vi "test-timer-all.vi"() -> (3 "ALL TESTS PASSED":bool)   [LabVIEW 2019]
uses:
  <vilib>/Rock Robotics/WPI/ThirdParty/JAS_Junk/TrajLib/Trajectory_Library.lvlib
panel:
  out "Expired 2":bool
  out "Expired":bool
  out "T2 After Start":dbl
  out "Passed 2":bool
  out "T1 After Stop":dbl
  out "T1 After Start":dbl
  out "Passed 0A":bool
  out "Passed 0":bool
  out "T0 - Diff = 5.0":dbl
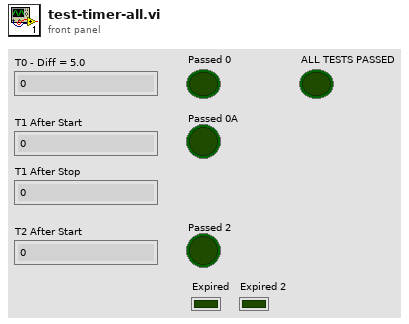
[diagram p1: front panel]
types:
  T1 = typedef "Trajectory_Library.lvlib/TIMER.ctl" = cluster{"StartTime":dbl, "Accumulated TIme":dbl, "Running":bool, "semaphore":T2}
  T2 = typedef "Semaphore RefNum" = refnum<k1>
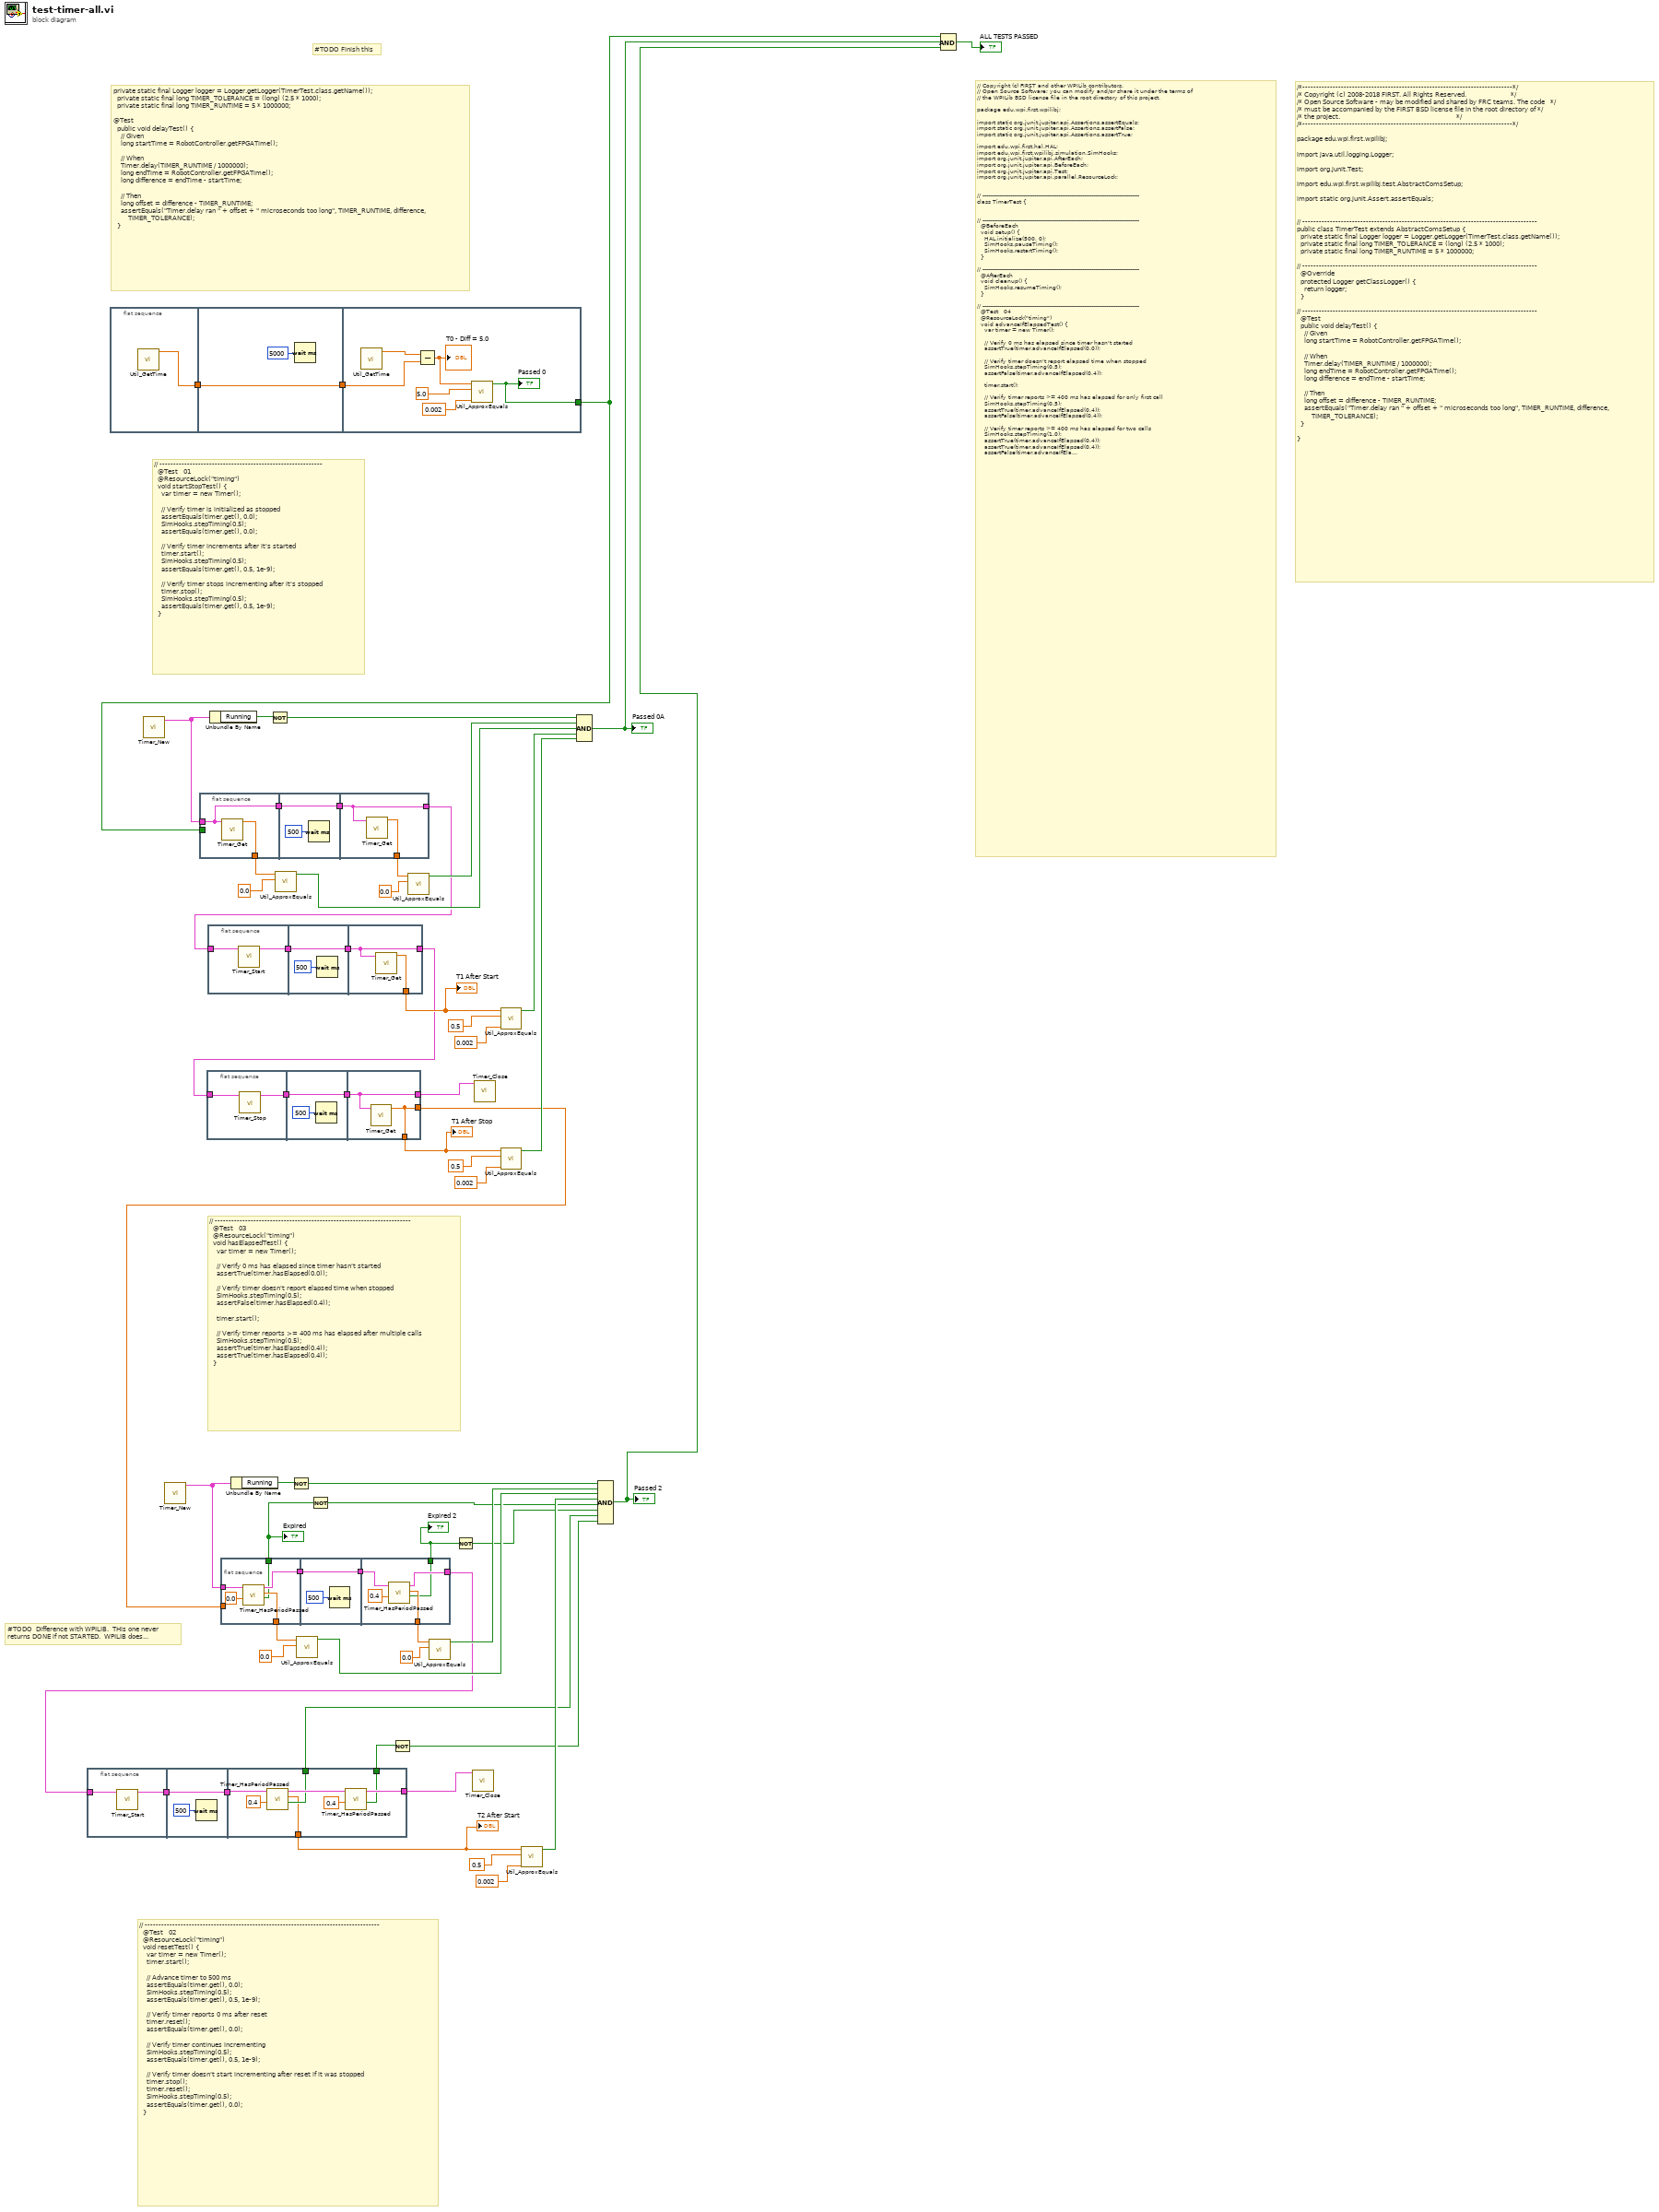
[diagram p0: block diagram]
diagram:
  # "#TODO Finish this"
  # "// -------------------------------------------------------------------------------------\n  @Test   02\n  @ResourceLock(\"timing\")\n  void resetTest() {\n    var timer = new Timer();\n    timer.start();\n\n    // Advance timer to 500 ms\n    assertEquals(timer.get(), 0.0);\n    SimHooks.stepTiming(0.5);\n    assertEquals(timer.get(), 0.5, 1e-9);\n\n    // Verify timer reports 0 ms after reset\n    timer.reset();\n    assertEquals(timer.get(), 0.0);\n\n    // Verify timer continues incrementing\n    SimHooks.stepTiming(0.5);\n    assertEquals(timer.get(), 0.5, 1e-9);\n\n    // Verify timer doesn't start incrementing after reset if it was stopped\n    timer.stop();\n    timer.reset();\n    SimHooks.stepTiming(0.5);\n    assertEquals(timer.get(), 0.0);\n  }"
  # "#TODO  Difference with WPILIB.  THis one never\nreturns DONE if not STARTED.  WPILIB does..."
  # "// -----------------------------------------------------------------------\n  @Test   03\n  @ResourceLock(\"timing\")\n  void hasElapsedTest() {\n    var timer = new Timer();\n\n    // Verify 0 ms has elapsed since timer hasn't started\n    assertTrue(timer.hasElapsed(0.0));\n\n    // Verify timer doesn't report elapsed time when stopped\n    SimHooks.stepTiming(0.5);\n    assertFalse(timer.hasElapsed(0.4));\n\n    timer.start();\n\n    // Verify timer reports >= 400 ms has elapsed after multiple calls\n    SimHooks.stepTiming(0.5);\n    assertTrue(timer.hasElapsed(0.4));\n    assertTrue(timer.hasElapsed(0.4));\n  }"
  # "// -----------------------------------------------------------\n  @Test   01\n  @ResourceLock(\"timing\")\n  void startStopTest() {\n    var timer = new Timer();\n\n    // Verify timer is initialized as stopped\n    assertEquals(timer.get(), 0.0);\n    SimHooks.stepTiming(0.5);\n    assertEquals(timer.get(), 0.0);\n\n    // Verify timer increments after it's started\n    timer.start();\n    SimHooks.stepTiming(0.5);\n    assertEquals(timer.get(), 0.5, 1e-9);\n\n    // Verify timer stops incrementing after it's stopped\n    timer.stop();\n    SimHooks.stepTiming(0.5);\n    assertEquals(timer.get(), 0.5, 1e-9);\n  }"
  # "/*----------------------------------------------------------------------------*/\n/* Copyright (c) 2008-2018 FIRST. All Rights Reserved.                        */\n/* Open Source Software - may be modified and shared by FRC teams. The code   */\n/* must be accompanied by the FIRST BSD license file in the root directory of */\n/* the project.                                                               */\n/*----------------------------------------------------------------------------*/\n\npackage edu.wpi.first.wpilibj;\n\nimport java.util.logging.Logger;\n\nimport org.junit.Test;\n\nimport edu.wpi.first.wpilibj.test.AbstractComsSetup;\n\nimport static org.junit.Assert.assertEquals;\n\n\n// -------------------------------------------------------------------------------------\npublic class TimerTest extends AbstractComsSetup {\n  private static final Logger logger = Logger.getLogger(TimerTest.class.getName());\n  private static final long TIMER_TOLERANCE = (long) (2.5 * 1000);\n  private static final long TIMER_RUNTIME = 5 * 1000000;\n\n// -------------------------------------------------------------------------------------\n  @Override\n  protected Logger getClassLogger() {\n    return logger;\n  }\n\n// -------------------------------------------------------------------------------------\n  @Test\n  public void delayTest() {\n    // Given\n    long startTime = RobotController.getFPGATime();\n\n    // When\n    Timer.delay(TIMER_RUNTIME / 1000000);\n    long endTime = RobotController.getFPGATime();\n    long difference = endTime - startTime;\n\n    // Then\n    long offset = difference - TIMER_RUNTIME;\n    assertEquals(\"Timer.delay ran \" + offset + \" microseconds too long\", TIMER_RUNTIME, difference,\n        TIMER_TOLERANCE);\n  }\n\n}"
  # "// Copyright (c) FIRST and other WPILib contributors.\n// Open Source Software; you can modify and/or share it under the terms of\n// the WPILib BSD license file in the root directory of this project.\n\npackage edu.wpi.first.wpilibj;\n\nimport static org.junit.jupiter.api.Assertions.assertEquals;\nimport static org.junit.jupiter.api.Assertions.assertFalse;\nimport static org.junit.jupiter.api.Assertions.assertTrue;\n\nimport edu.wpi.first.hal.HAL;\nimport edu.wpi.first.wpilibj.simulation.SimHooks;\nimport org.junit.jupiter.api.AfterEach;\nimport org.junit.jupiter.api.BeforeEach;\nimport org.junit.jupiter.api.Test;\nimport org.junit.jupiter.api.parallel.ResourceLock;\n\n\n// -------------------------------------------------------------------------------------\nclass TimerTest {\n\n\n// -------------------------------------------------------------------------------------\n  @BeforeEach\n  void setup() {\n    HAL.initialize(500, 0);\n    SimHooks.pauseTiming();\n    SimHooks.restartTiming();\n  }\n\n// -------------------------------------------------------------------------------------\n  @AfterEach\n  void cleanup() {\n    SimHooks.resumeTiming();\n  }\n\n// -------------------------------------------------------------------------------------\n  @Test   04\n  @ResourceLock(\"timing\")\n  void advanceIfElapsedTest() {\n    var timer = new Timer();\n\n    // Verify 0 ms has elapsed since timer hasn't started\n    assertTrue(timer.advanceIfElapsed(0.0));\n\n    // Verify timer doesn't report elapsed time when stopped\n    SimHooks.stepTiming(0.5);\n    assertFalse(timer.advanceIfElapsed(0.4));\n\n    timer.start();\n\n    // Verify timer reports >= 400 ms has elapsed for only first call\n    SimHooks.stepTiming(0.5);\n    assertTrue(timer.advanceIfElapsed(0.4));\n    assertFalse(timer.advanceIfElapsed(0.4));\n\n    // Verify timer reports >= 400 ms has elapsed for two calls\n    SimHooks.stepTiming(1.0);\n    assertTrue(timer.advanceIfElapsed(0.4));\n    assertTrue(timer.advanceIfElapsed(0.4));\n    assertFalse(timer.advanceIfElapsed(0.4));\n  }\n\n// -------------------------------------------------------------------------------------\n  @Test   05\n  @ResourceLock(\"timing\")\n  void getFPGATimestampTest() {\n    double start = Timer.getFPGATimestamp();\n    SimHooks.stepTiming(0.5);\n    double end = Timer.getFPGATimestamp();\n    assertEquals(start + 0.5, end, 1e-9);\n\n\n  }\n}"
  # "private static final Logger logger = Logger.getLogger(TimerTest.class.getName());\n  private static final long TIMER_TOLERANCE = (long) (2.5 * 1000);\n  private static final long TIMER_RUNTIME = 5 * 1000000;\n\n@Test\n  public void delayTest() {\n    // Given\n    long startTime = RobotController.getFPGATime();\n\n    // When\n    Timer.delay(TIMER_RUNTIME / 1000000);\n    long endTime = RobotController.getFPGATime();\n    long difference = endTime - startTime;\n\n    // Then\n    long offset = difference - TIMER_RUNTIME;\n    assertEquals(\"Timer.delay ran \" + offset + \" microseconds too long\", TIMER_RUNTIME, difference,\n        TIMER_TOLERANCE);\n  }"
  n1 = flat-sequence {
    tunnel: w19 -> [w61]
    tunnel: [w60] -> w29
    tunnel: [w62] -> w28
    tunnel: w29 -> [w62]
    tunnel: [w64] -> w17
    tunnel: w28 -> [w71]
    tunnel: [w69] -> w5
    tunnel: [w66] -> w8
    tunnel: [w65] -> w7
    frame #0 {
      n2 = call <vilib>:"Timer_Start.vi"("in Timer"=w61) -> ("out Timer"=w60:T1)  [unwired: 10 in]
    }
    frame #1 {
      n3 = Wait (ms)(milliseconds to wait=u32 500) -> ()  [unwired: 1 out]
    }
    frame #2 {
      n4 = call <vilib>:"Timer_HasPeriodPassed.vi"("Period"=0.4, "in Timer"=w71) -> ("Expired"=w66:bool, "CurrentTImer"=w64:dbl, "out Timer"=w70:T1)  [unwired: 7 in]
      n5 = call <vilib>:"Timer_HasPeriodPassed.vi"("Period"=0.4, "in Timer"=w70) -> ("Expired"=w65:bool, "out Timer"=w69:T1)  [unwired: 7 in, 1 out]
    }
  }
  n6 = flat-sequence {
    tunnel: [w72] -> w59
    tunnel: [w73] -> w58
    tunnel: w59 -> [w73]
    tunnel: w58 -> [w79]
    tunnel: [w75] -> w2
    frame #0 {
      n7 = call <vilib>:"Util_GetTime.vi"() -> ("FPGA_Time_Seconds"=w72:dbl)  [unwired: 10 in, 1 out]
    }
    frame #1 {
      n8 = Wait (ms)(milliseconds to wait=u32 5000) -> ()  [unwired: 1 out]
    }
    frame #2 {
      n9 = call <vilib>:"Util_GetTime.vi"() -> ("FPGA_Time_Seconds"=w80:dbl)  [unwired: 10 in, 1 out]
      n10 = Subtract(x=w80, y=w79) -> (x-y=w78:dbl)
      "T0 - Diff = 5.0" <- w78
      n11 = call "Util_ApproxEquals.vi"("Tolerance"=0.002, "Value 2"=5.0, "Value 1"=w78) -> ("ApproxEquals"=w75:bool)  [unwired: 8 in]
      "Passed 0" <- w75
    }
  }
  n12 = call <vilib>:"Timer_New.vi"() -> ("TIMER"=w55:T1)  [unwired: 11 in]
  n13 = call <vilib>:"Timer_New.vi"() -> ("TIMER"=w25:T1)  [unwired: 11 in]
  n14 = flat-sequence {
    tunnel: w55 -> [w81]
    tunnel: [w82] -> w53
    tunnel: [w81] -> w47
    tunnel: w2 -> [_]
    tunnel: [w83] -> w48
    tunnel: w47 -> [w83]
    tunnel: [w86] -> w54
    tunnel: w48 -> [w85]
    tunnel: [w85] -> w46
    frame #0 {
      n15 = call <vilib>:"Timer_Get.vi"("TIMER"=w81) -> ("CurrentTImer"=w82:dbl)  [unwired: 10 in]
    }
    frame #1 {
      n16 = Wait (ms)(milliseconds to wait=u32 500) -> ()  [unwired: 1 out]
    }
    frame #2 {
      n17 = call <vilib>:"Timer_Get.vi"("TIMER"=w85) -> ("CurrentTImer"=w86:dbl)  [unwired: 10 in]
    }
  }
  n18 = flat-sequence {
    tunnel: [w87] -> w39
    tunnel: w37 -> [w88]
    tunnel: [w89] -> w38
    tunnel: w39 -> [w89]
    tunnel: [w91] -> w33
    tunnel: w38 -> [w92]
    tunnel: [w92] -> w32
    tunnel: [w91] -> w14
    frame #0 {
      n19 = call <vilib>:"Timer_Stop.vi"("in Timer"=w88) -> ("out Timer"=w87:T1)  [unwired: 10 in]
    }
    frame #1 {
      n20 = Wait (ms)(milliseconds to wait=u32 500) -> ()  [unwired: 1 out]
    }
    frame #2 {
      n21 = call <vilib>:"Timer_Get.vi"("TIMER"=w92) -> ("CurrentTImer"=w91:dbl)  [unwired: 10 in]
    }
  }
  n22 = flat-sequence {
    tunnel: w46 -> [w94]
    tunnel: [w93] -> w44
    tunnel: [w95] -> w45
    tunnel: w44 -> [w95]
    tunnel: [w98] -> w42
    tunnel: w45 -> [w97]
    tunnel: [w97] -> w37
    frame #0 {
      n23 = call <vilib>:"Timer_Start.vi"("in Timer"=w94) -> ("out Timer"=w93:T1)  [unwired: 10 in]
    }
    frame #1 {
      n24 = Wait (ms)(milliseconds to wait=u32 500) -> ()  [unwired: 1 out]
    }
    frame #2 {
      n25 = call <vilib>:"Timer_Get.vi"("TIMER"=w97) -> ("CurrentTImer"=w98:dbl)  [unwired: 10 in]
    }
  }
  n26 = Unbundle By Name(w55) -> ("Running"=w57:bool)
  n27 = flat-sequence {
    tunnel: w25 -> [w102]
    tunnel: [w103] -> w24
    tunnel: [w100] -> w31
    tunnel: w14 -> [_]
    tunnel: [w99] -> w10
    tunnel: [w104] -> w30
    tunnel: w31 -> [w104]
    tunnel: w30 -> [w110]
    tunnel: [w109] -> w19
    tunnel: [w107] -> w13
    tunnel: [w106] -> w12
    frame #0 {
      n28 = call <vilib>:"Timer_HasPeriodPassed.vi"("Period"=0.0, "in Timer"=w102) -> ("Expired"=w99:bool, "CurrentTImer"=w103:dbl, "out Timer"=w100:T1)  [unwired: 7 in]
    }
    frame #1 {
      n29 = Wait (ms)(milliseconds to wait=u32 500) -> ()  [unwired: 1 out]
    }
    frame #2 {
      n30 = call <vilib>:"Timer_HasPeriodPassed.vi"("Period"=0.4, "in Timer"=w110) -> ("Expired"=w106:bool, "CurrentTImer"=w107:dbl, "out Timer"=w109:T1)  [unwired: 7 in]
    }
  }
  n31 = Unbundle By Name(w25) -> ("Running"=w27:bool)
  n32 = Not(x=w57) -> (.not. x?=w56:bool)
  n33 = call "Util_ApproxEquals.vi"("Value 2"=0.0, "Value 1"=w53) -> ("ApproxEquals"=w49:bool)  [unwired: 9 in]
  n34 = Not(x=w27) -> (.not. x?=w26:bool)
  n35 = call "Util_ApproxEquals.vi"("Value 2"=0.0, "Value 1"=w24) -> ("ApproxEquals"=w20:bool)  [unwired: 9 in]
  n36 = Not(x=w10) -> (.not. x?=w11:bool)
  n37 = Not(x=w7) -> (.not. x?=w6:bool)
  n38 = call "Util_ApproxEquals.vi"("Value 2"=0.0, "Value 1"=w54) -> ("ApproxEquals"=w50:bool)  [unwired: 9 in]
  n39 = call "Util_ApproxEquals.vi"("Value 2"=0.0, "Value 1"=w13) -> ("ApproxEquals"=w21:bool)  [unwired: 9 in]
  n40 = Not(x=w12) -> (.not. x?=w9:bool)
  n41 = call <vilib>:"Timer_Close.vi"("TIMER"=w5) -> ()  [unwired: 11 in]
  n42 = call <vilib>:"Timer_Close.vi"("TIMER"=w32) -> ()  [unwired: 11 in]
  n43 = call "Util_ApproxEquals.vi"("Tolerance"=0.002, "Value 2"=0.5, "Value 1"=w42) -> ("ApproxEquals"=w41:bool)  [unwired: 8 in]
  n44 = call "Util_ApproxEquals.vi"("Tolerance"=0.002, "Value 2"=0.5, "Value 1"=w33) -> ("ApproxEquals"=w34:bool)  [unwired: 8 in]
  n45 = call "Util_ApproxEquals.vi"("Tolerance"=0.002, "Value 2"=0.5, "Value 1"=w17) -> ("ApproxEquals"=w16:bool)  [unwired: 8 in]
  n46 = Compound Arithmetic op=AND(w56, w50, w49, w41, w34) -> (w3:bool)
  "Passed 0A" <- w3
  n47 = Compound Arithmetic op=AND(w26, w21, w20, w16, w11, w9, w8, w6) -> (w1:bool)
  "Passed 2" <- w1
  n48 = Compound Arithmetic op=AND(w2, w3, w1) -> (→"ALL TESTS PASSED":bool)
  "T1 After Start" <- w42
  "T1 After Stop" <- w33
  "T2 After Start" <- w17
  "Expired" <- w10
  "Expired 2" <- w12
